vi "ReadAttributeFast.vi"(0 "reference in":refnum<class "TestClass.lvclass">, 5 "error in (no error)":errorcluster) -> (14 "reference out":refnum<class "TestClass.lvclass">, 16 "SingleData":dbl, 19 "error out":errorcluster)   [LabVIEW 2017, in "TestClass.lvclass"]
doc: "Reads the attributes with high performance."
uses:
  TestClass.lvclass
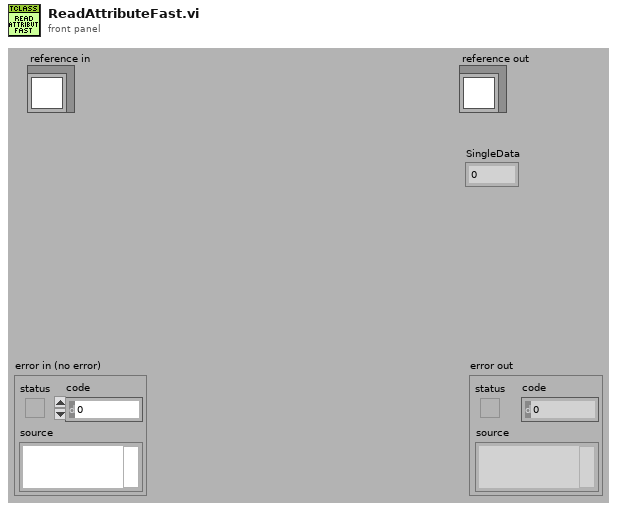
[diagram p1: front panel]
types:
  T1 = typedef "TestClass.lvclass/ObjectAttributesRef.ctl" = refnum<data-value>
  T2 = typedef "TestClass.lvclass/ObjectAttributes.ctl" = cluster{"SingleData":dbl, "LargeData":dbl[]}
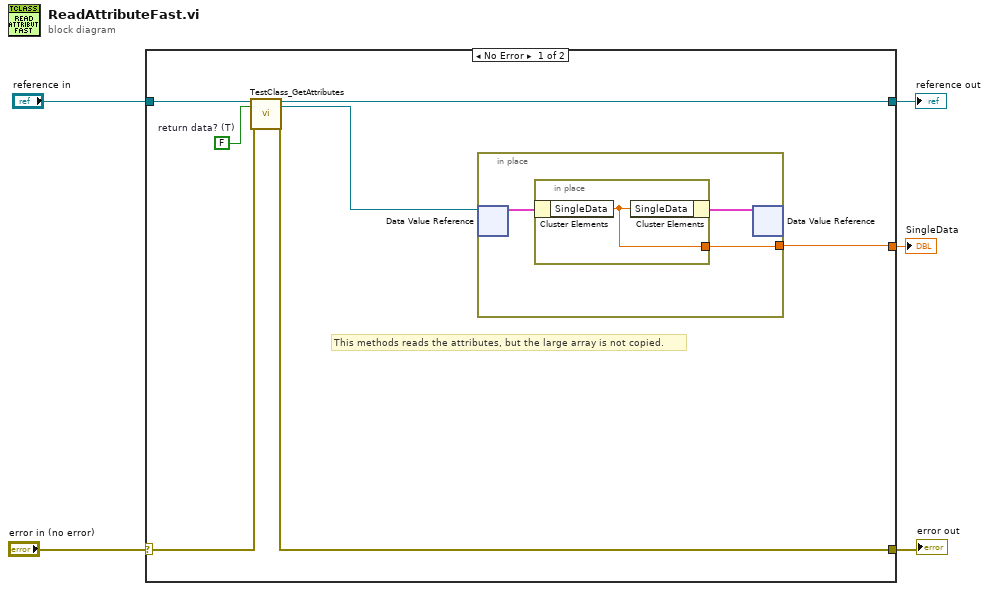
[diagram p0: block diagram]
diagram:
  n1 = case shown="No Error" "error in (no error)" {
    selector: "error in (no error)" -> [w12 w18]
    tunnel: [w11 w18] -> w4
    tunnel: [w9 w17] -> w2
    tunnel: "reference in" -> [w10 w17]
    tunnel: [w6 _] -> w1
    frame No Error {
      w8 = FALSE  # return data? (T)
      # "This methods reads the attributes, but the large array is not copied."
      n2 = call "TestClass_GetAttributes.vi"("reference in"=w10, "return data? (T)"=w8, "error in (no error)"=w12) -> ("reference out"=w9:refnum<class "TestClass.lvclass">, "attributes ref"=w7:T1, "error out"=w11:errorcluster)  [unwired: 13 in, 1 out]
      n3 = in-place {
        in-place-border: [w13] -> w6
        n4 = in-place-dvr #1(w7) -> (w15:T2)  [unwired: 1 out]
        n5 = in-place {
          in-place-border: [w16] -> w13
          n6 = in-place-cluster #2(w15) -> ("SingleData"=w16:dbl)
          n7 = in-place-cluster #2("SingleData"=w16) -> (w14:T2)
        }
        n8 = in-place-dvr #1(w14) -> ()  [unwired: 2 out]
      }
    }
    frame Error {
    }
  }
  "error out" <- w4
  "reference out" <- w2
  "SingleData" <- w1
